vi "libdaq_device_get_count.vi"(0 "error in (no error)":errorcluster) -> (14 "error out":errorcluster, 17 "device_count":i32)   [LabVIEW 2010, in "libdaqVI.lvlib"]
doc: "获取连接到计算机系统上的DAQ设备的数量"
uses:
  libdaqVI.lvlib
  dll/daqlib.dll
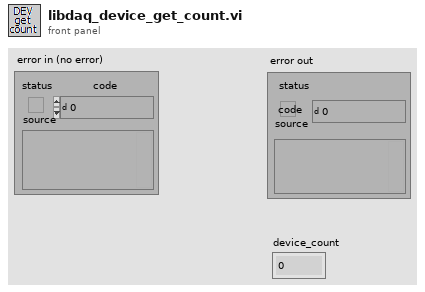
[diagram p1: front panel]
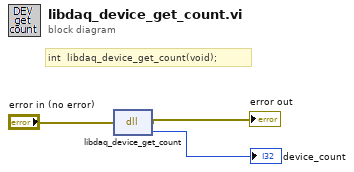
[diagram p0: block diagram]
diagram:
  # "int  libdaq_device_get_count(void);"
  n1 = dll-call lib="E:/Product/Example/DAQ-USB3212/Labview/labview_2010/libdaqVI/dll/daqlib.dll" fn="libdaq_device_get_count"(error in="error in (no error)") -> (error out=→"error out":errorcluster, "return type"=→"device_count":i32)  [unwired: 2 in, 1 out]
